vi "NanoDriveInfo-SubVI.vi"(0 "Handle":i32) -> (8 "ADC resolution (bits)":i16, 10 "DAC resolution (bits)":i16, 12 "Product ID (in hex)":string, 13 "Serial #":i32, 14 "Firmware Version":i16, 15 "DAC Freq (ms)":dbl format="%.4f", 16 "Firmware Profile":i16, 17 "ADC Freq (ms)":dbl format="%.4f", 18 "Dll Version":i16, 19 "Dll Revision":i16, 20 "X axis":bool, 21 "Y axis":bool, 22 "Z axis":bool, 23 "Aux axis":bool, 24 "X Calibration":dbl caption="Calibration (um)" format="%.3f", 25 "Y Calibration":dbl format="%.3f", 26 "Z Calibration":dbl format="%.3f", 27 "Aux Calibration":dbl format="%.3f")   [LabVIEW 2014]
uses:
  Library Files - Andor and MadCity/Madlib/Madlib.dll
panel:
  # "This example VI provides access to (and demonstrates how to access)\n important device information."
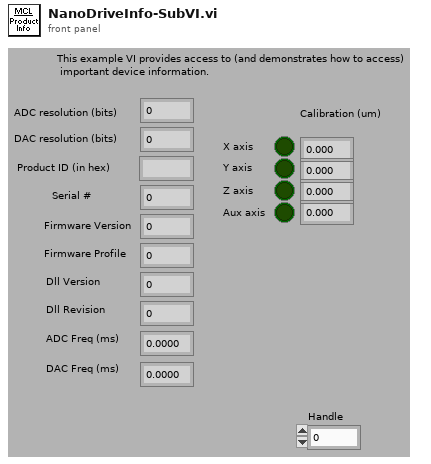
[diagram p1: front panel]
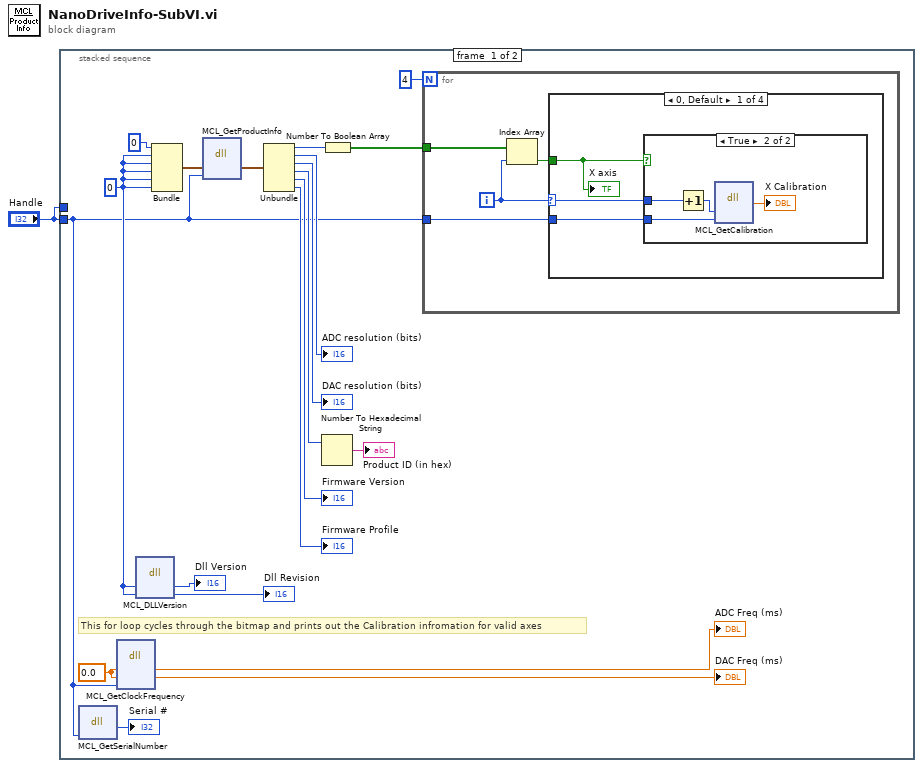
[diagram p0: block diagram]
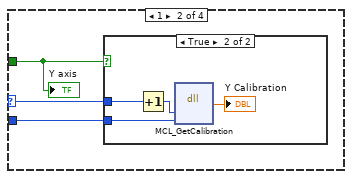
[diagram p3: hidden frame]
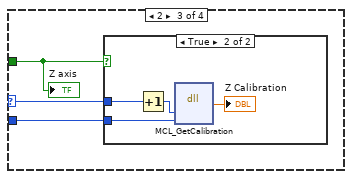
[diagram p5: hidden frame]
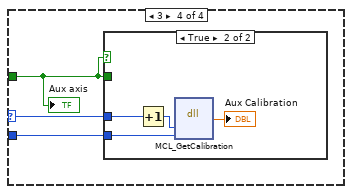
[diagram p7: hidden frame]
diagram:
  n1 = stacked-sequence {
    tunnel: "Handle" -> [w2 _]
    tunnel: "Handle" -> [_ _]
    frame #0 {
      w9 = 0.0
      w12 = i16 0
      # "This for loop cycles through the bitmap and prints out the Calibration infromation for valid axes"
      n2 = dll-call lib="C:/Users/Bakir/Desktop/LabFiles/Testing/Library Files - Andor and MadCity/Madlib/Madlib.dll" fn="MCL_GetSerialNumber"("handle"=w2) -> ("return type"=→"Serial #":i32)  [unwired: 4 in, 2 out]
      n3 = dll-call lib="C:/Users/Bakir/Desktop/LabFiles/Testing/Library Files - Andor and MadCity/Madlib/Madlib.dll" fn="MCL_GetClockFrequency"("ADC freq"=w9, "DAC freq"=w9, "handle"=w2) -> ("ADC freq"=→"ADC Freq (ms)":dbl, "DAC freq"=→"DAC Freq (ms)":dbl)  [unwired: 4 in, 3 out]
      n4 = dll-call lib="C:/Users/Bakir/Desktop/LabFiles/Testing/Library Files - Andor and MadCity/Madlib/Madlib.dll" fn="MCL_DLLVersion"("version"=w12, "revision"=w12) -> ("version"=→"Dll Version":i16, "revision"=→"Dll Revision":i16)  [unwired: 3 in, 3 out]
      n5 = Bundle(u8 0, w12, w12, w12, w12, w12) -> (w20:cluster{u8, i16, i16, i16, i16, i16})  [unwired: 1 out]
      n6 = dll-call lib="C:/Users/Bakir/Desktop/LabFiles/Testing/Library Files - Andor and MadCity/Madlib/Madlib.dll" fn="MCL_GetProductInfo"("ProductInformation"=w20, "handle"=w2) -> ("ProductInformation"=w19:cluster{u8, i16, i16, i16, i16, i16})  [unwired: 4 in, 3 out]
      n7 = Unbundle(w19) -> (w6:u8, →"ADC resolution (bits)":i16, →"DAC resolution (bits)":i16, w18:i16, →"Firmware Version":i16, →"Firmware Profile":i16)
      n8 = Number To Hexadecimal String(2:w18) -> (0:→"Product ID (in hex)":string)  [unwired: 1 out]
      n9 = Number To Boolean Array(number=w6) -> (Boolean array=w5:bool[])
      n10 = for {
        N: 4 -> [_]
        tunnel: w5 -> [w25]
        tunnel: w2 -> [w22]
        i -> [w24]
        n11 = Index Array(array=w25, index=w24) -> (element=w23:bool)
        n12 = case shown="0, Default" w24 {
          selector: w24 -> [w28 w35 w42 w49]
          tunnel: w23 -> [w27 w34 w41 w48]
          tunnel: w22 -> [w26 w33 w40 w47]
          frame 0, Default {
            n13 = case shown="True" w27 {
              tunnel: w28 -> [_ w32]
              tunnel: w26 -> [_ w29]
              frame False {
              }
              frame True {
                n14 = Increment(x=w32) -> (x+1=w30:i32)
                n15 = dll-call lib="C:/Users/Bakir/Desktop/LabFiles/Testing/Library Files - Andor and MadCity/Madlib/Madlib.dll" fn="MCL_GetCalibration"("axis"=w30, "handle"=w29) -> ("return type"=→"X Calibration":dbl)  [unwired: 5 in, 2 out]
              }
            }
            "X axis" <- w27
          }
          frame 1 {
            n16 = case shown="True" w34 {
              tunnel: w35 -> [_ w39]
              tunnel: w33 -> [_ w37]
              frame False {
              }
              frame True {
                n17 = Increment(x=w39) -> (x+1=w38:i32)
                n18 = dll-call lib="C:/Users/Bakir/Desktop/LabFiles/Testing/Library Files - Andor and MadCity/Madlib/Madlib.dll" fn="MCL_GetCalibration"("axis"=w38, "handle"=w37) -> ("return type"=→"Y Calibration":dbl)  [unwired: 5 in, 2 out]
              }
            }
            "Y axis" <- w34
          }
          frame 2 {
            n19 = case shown="True" w41 {
              tunnel: w42 -> [_ w46]
              tunnel: w40 -> [_ w44]
              frame False {
              }
              frame True {
                n20 = Increment(x=w46) -> (x+1=w43:i32)
                n21 = dll-call lib="C:/Users/Bakir/Desktop/LabFiles/Testing/Library Files - Andor and MadCity/Madlib/Madlib.dll" fn="MCL_GetCalibration"("axis"=w43, "handle"=w44) -> ("return type"=→"Z Calibration":dbl)  [unwired: 5 in, 2 out]
              }
            }
            "Z axis" <- w41
          }
          frame 3 {
            n22 = case shown="True" w48 {
              tunnel: w49 -> [_ w53]
              tunnel: w48 -> [_ _]
              tunnel: w47 -> [_ w50]
              frame False {
              }
              frame True {
                n23 = Increment(x=w53) -> (x+1=w51:i32)
                n24 = dll-call lib="C:/Users/Bakir/Desktop/LabFiles/Testing/Library Files - Andor and MadCity/Madlib/Madlib.dll" fn="MCL_GetCalibration"("axis"=w51, "handle"=w50) -> ("return type"=→"Aux Calibration":dbl)  [unwired: 5 in, 2 out]
              }
            }
            "Aux axis" <- w48
          }
        }
      }
    }
    frame #1 {
    }
  }
